vi "Strting 1D to Data Type.vi"(8 "error in (no error)":errorcluster, 11 "String 1D":string[](array[string])) -> (0 "error out":errorcluster, 3 "Boolean out":refnum<class "String 1D.lvclass">)   [LabVIEW 2017, in "String 1D.lvclass"]
uses:
  <vilib>/gpm_packages/@cs/data-type-serializer/source/String 1D/String 1D.lvclass
  <vilib>/gpm_packages/@cs/data-type-serializer/source/String 1D/String 1D.lvclass/String 1D.ctl
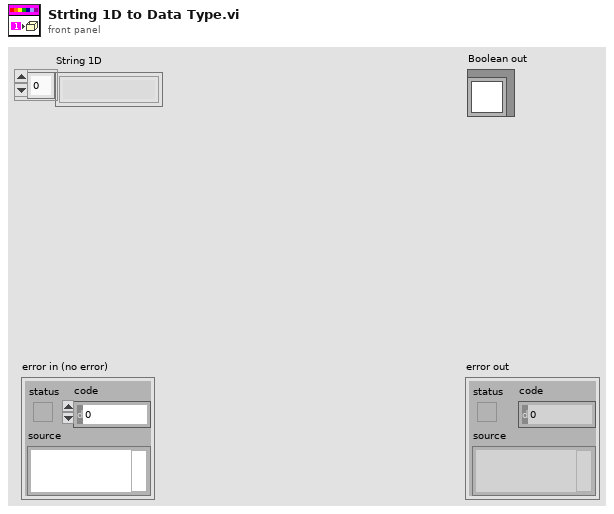
[diagram p1: front panel]
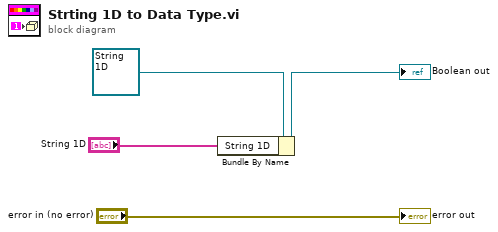
[diagram p0: block diagram]
diagram:
  n1 = Bundle By Name(cluster=refnum<class "String 1D.lvclass"> refnum ("Boolean in"), "String 1D"="String 1D") -> (→"Boolean out":refnum<class "String 1D.lvclass">)
  "error out" <- "error in (no error)"
